vi "EditorPopUp.vi"(8 "error in (no error)":errorcluster, 11 "MAUI.Editor":refnum<class "MAUI.Editor.lvclass">) -> (0 "error out":errorcluster, 3 "MAUI.Editor out":refnum<class "MAUI.Editor.lvclass">)   [LabVIEW 2019, in "MAUI.Editor.lvclass"]
uses:
  MAUI.Editor.lvclass
panel:
  in  "Listbox":i32(listbox)
  in  "Save":bool
  in  "Select":bool
  in  "Refresh":bool
  in  "Configure":bool
  in  "New":bool
  in  "Delete":bool
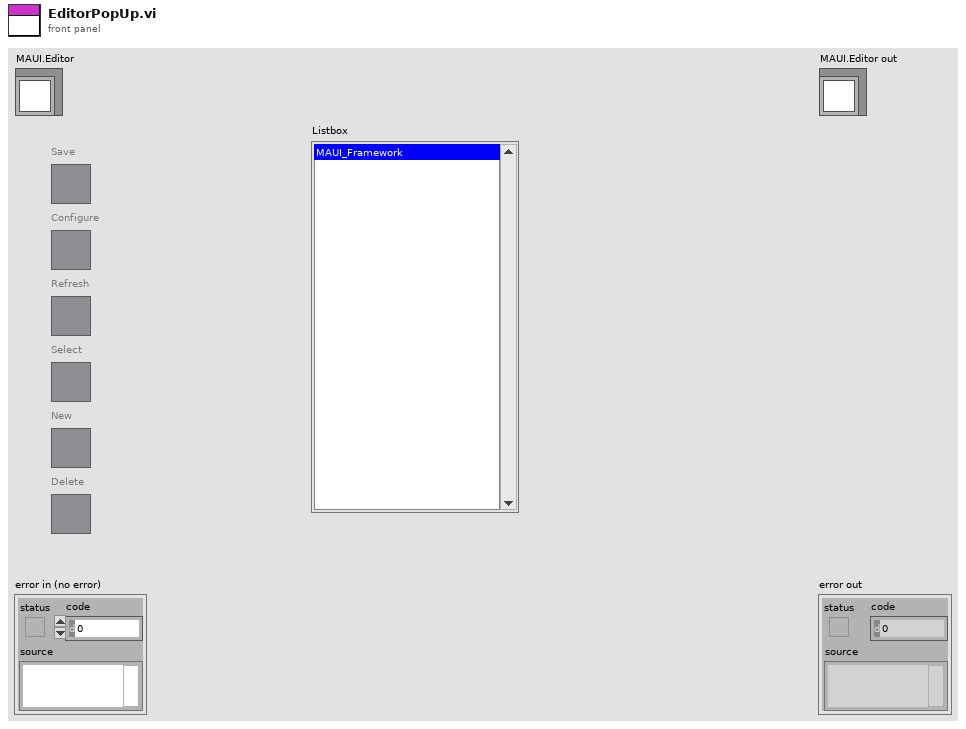
[diagram p1: front panel]
types:
  T1 = enum32{"Invalid", "Standard", "Closed", "Hidden", "Minimized", "Maximized"}
  T2 = enum32{"invalid app kind", "Development System", "Run Time System", "Student Edition", "Embedded LabVIEW", "Evaluation", "Custom"}
  T3 = cluster{"Core":cluster{"Current VI Reference":refnum<vi>, "Close Panel on Exit?":bool}, "MAUI.Editor":refnum<class "MAUI.Editor.lvclass">, "Unsaved?":bool}
  T4 = cluster{"Current VI Reference":refnum<vi>, "Close Panel on Exit?":bool}
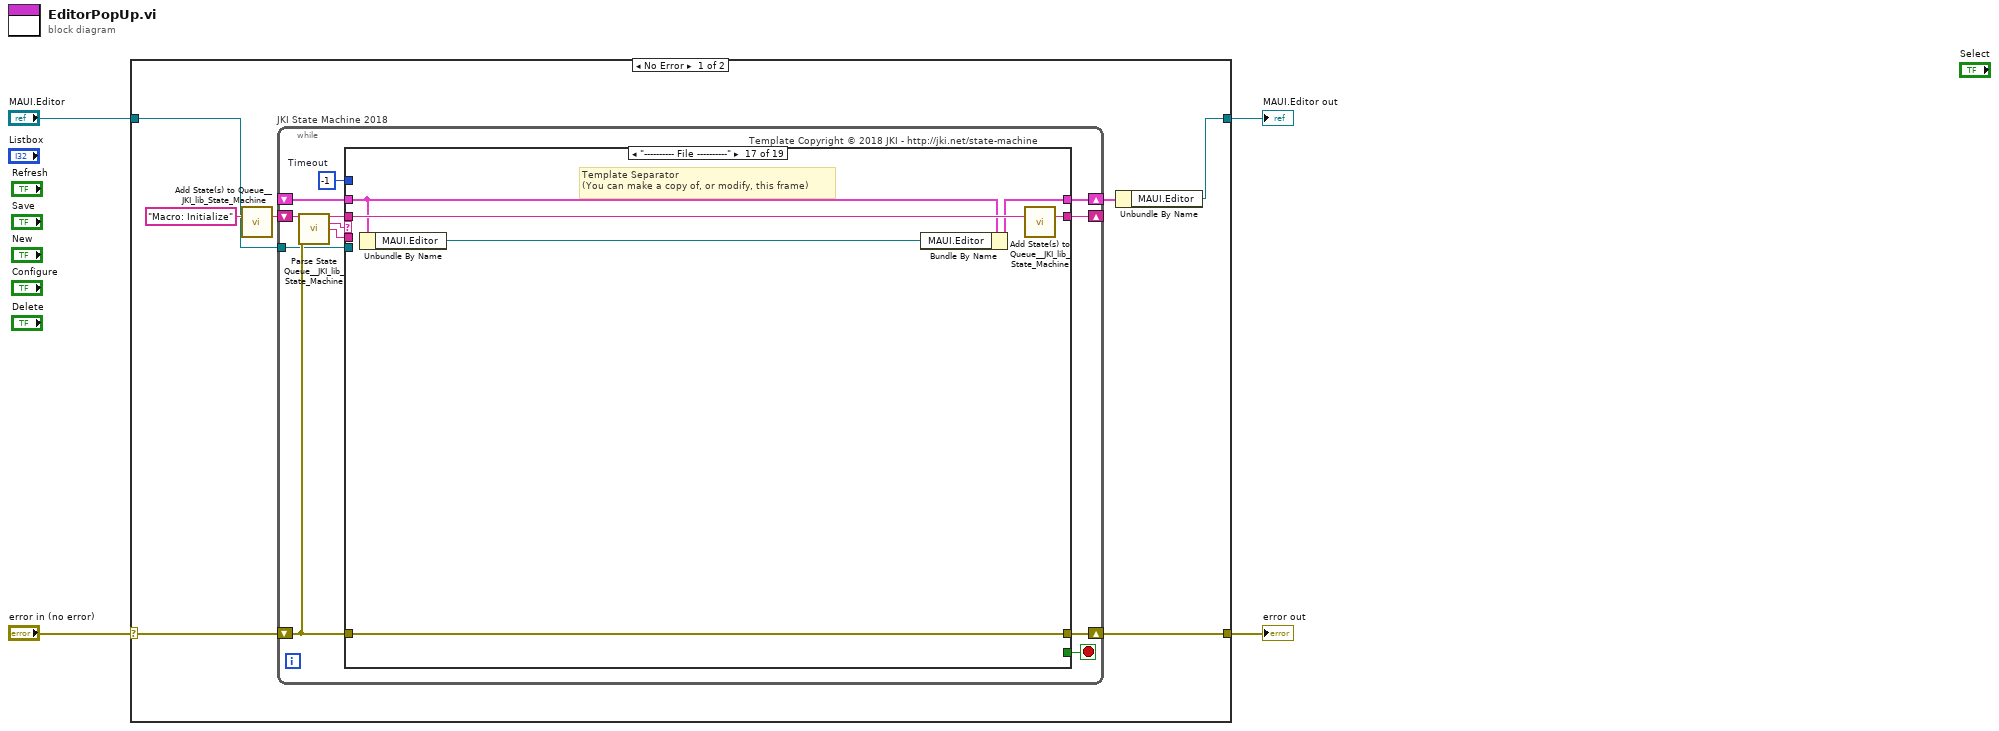
[diagram p0: block diagram]
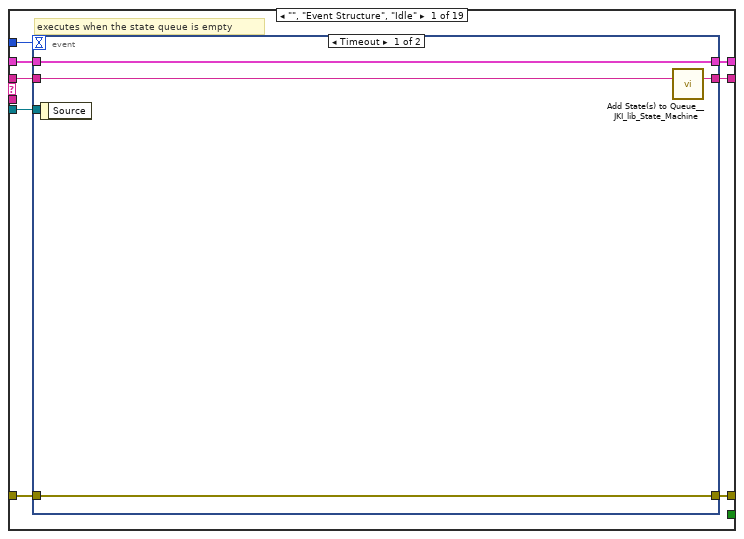
[diagram p2: hidden frame]
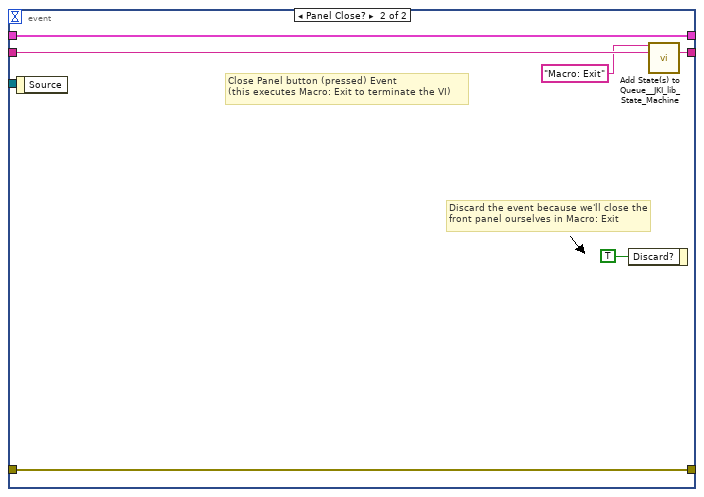
[diagram p3: hidden frame]
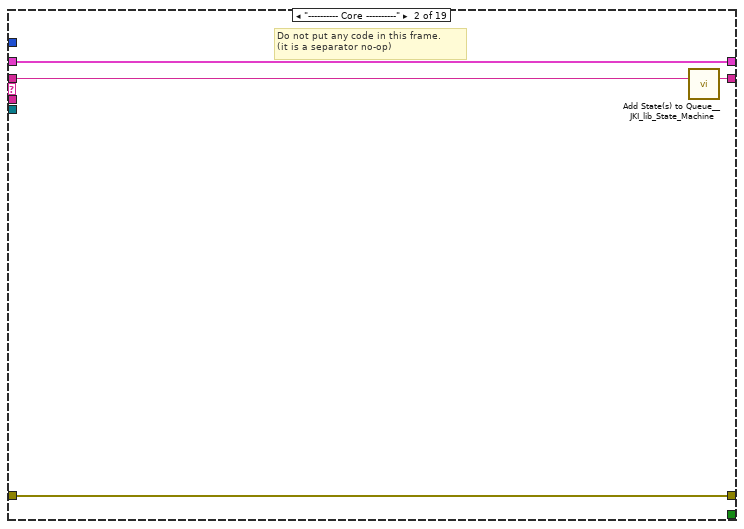
[diagram p4: hidden frame]
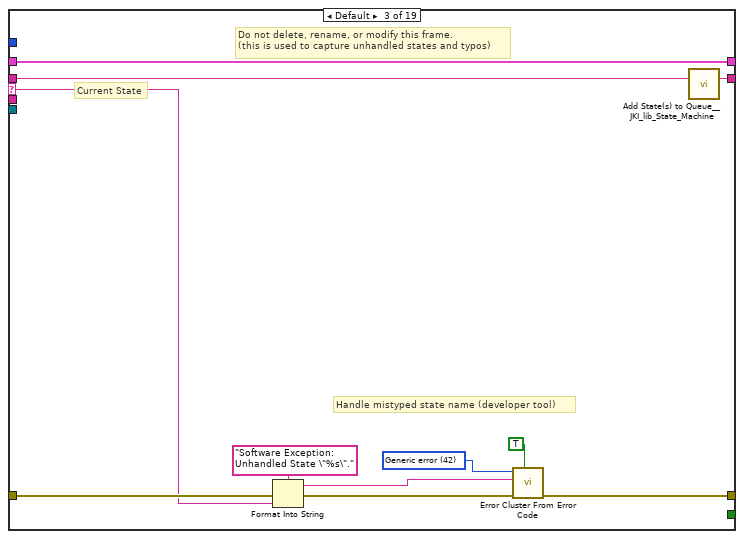
[diagram p5: hidden frame]
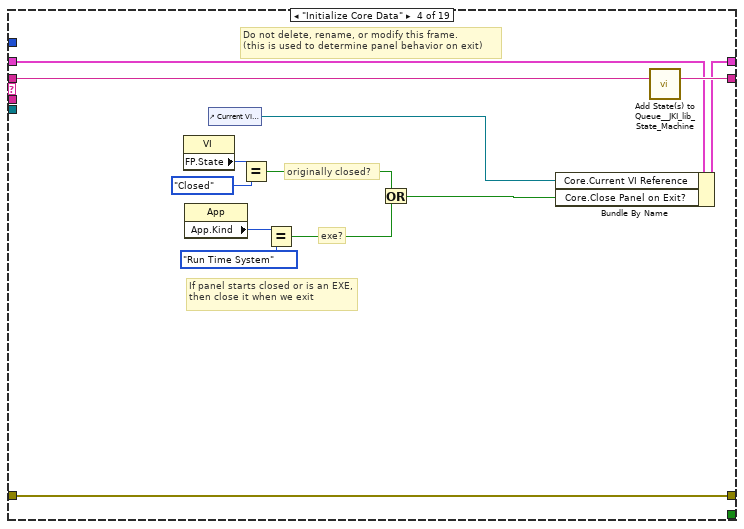
[diagram p6: hidden frame]
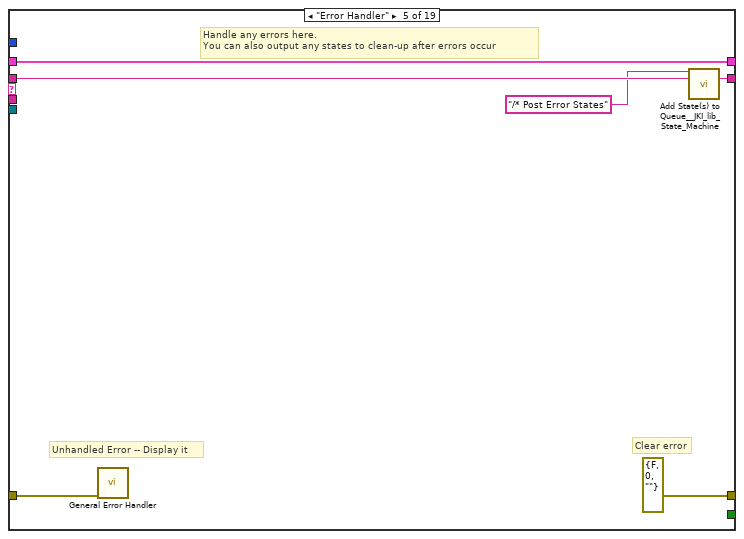
[diagram p7: hidden frame]
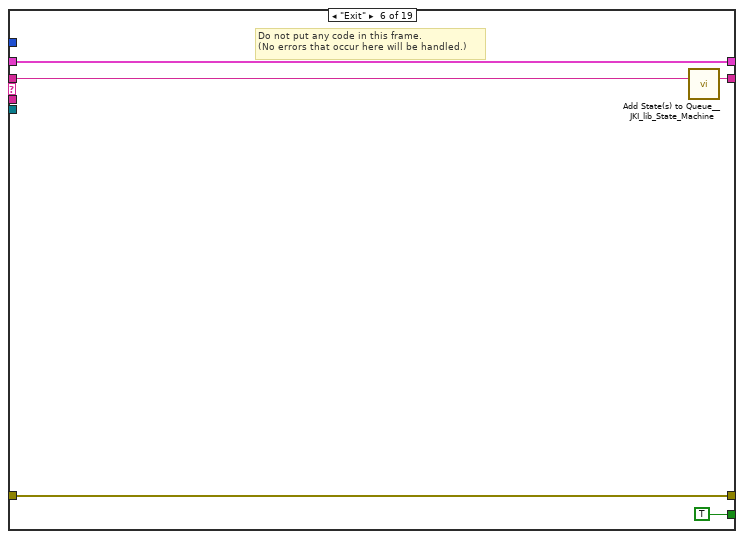
[diagram p8: hidden frame]
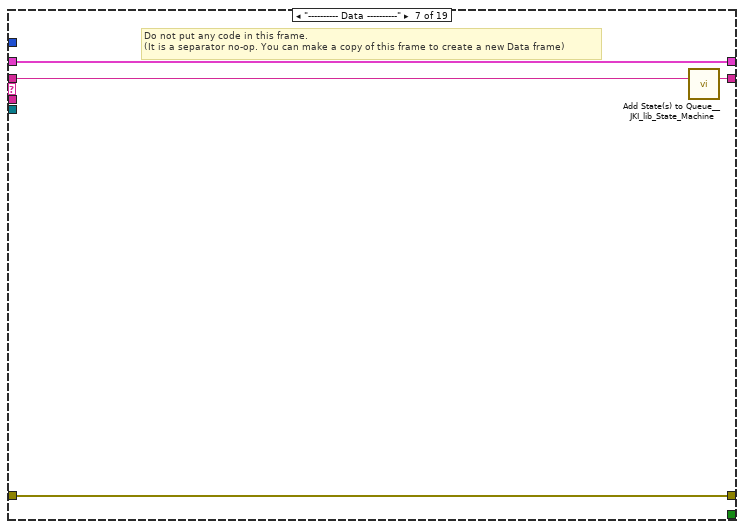
[diagram p9: hidden frame]
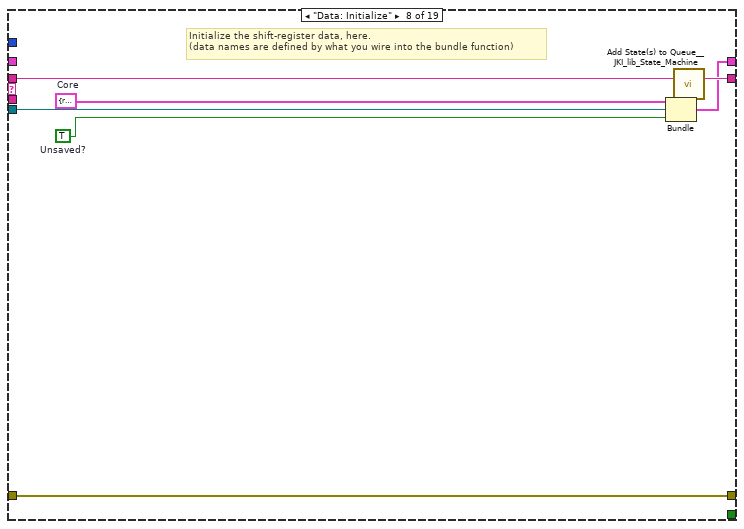
[diagram p10: hidden frame]
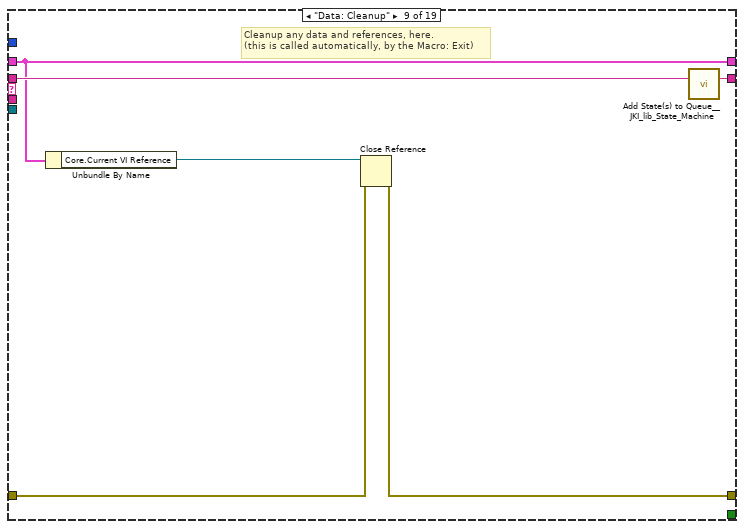
[diagram p11: hidden frame]
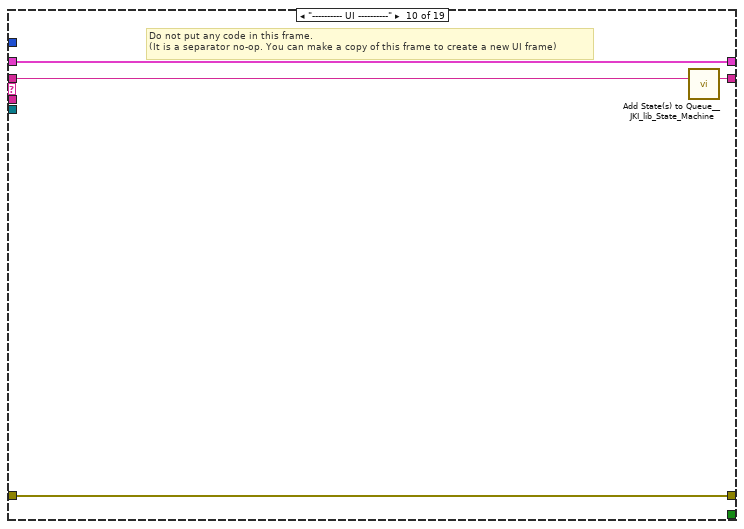
[diagram p12: hidden frame]
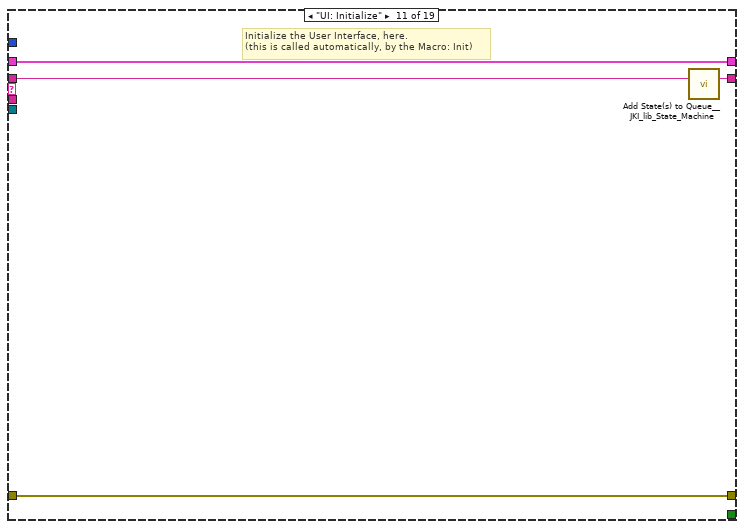
[diagram p13: hidden frame]
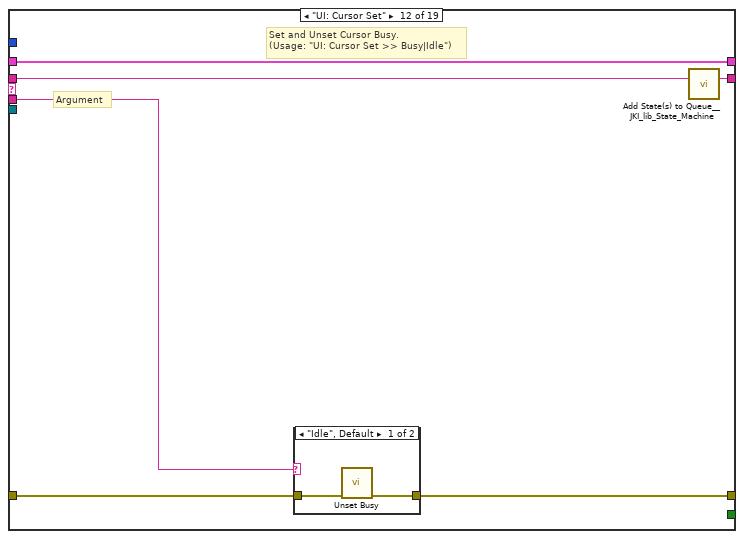
[diagram p14: hidden frame]
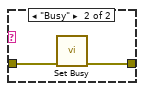
[diagram p15: hidden frame]
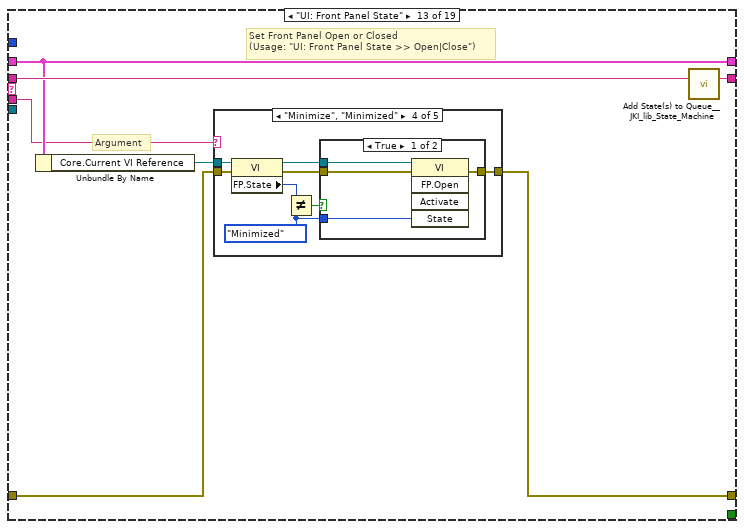
[diagram p16: hidden frame]
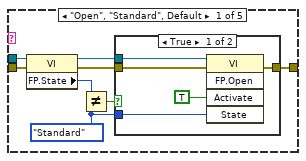
[diagram p17: hidden frame]
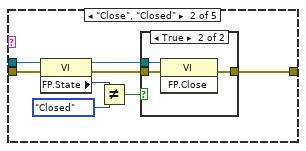
[diagram p19: hidden frame]
diagram:
  n1 = case shown="No Error" "error in (no error)" {
    selector: "error in (no error)" -> [w5 w224]
    tunnel: [w6 w224] -> w3
    tunnel: [w7 w223] -> w1
    tunnel: "MAUI.Editor" -> [w8 w223]
    frame No Error {
      n2 = call <vilib>:"Add State(s) to Queue__JKI_lib_State_Machine.vi"("State(s) in (\"\")"="Macro: Initialize") -> ("States Out"=w11:string)  [unwired: 14 in]
      n3 = while "JKI State Machine 2018" {
        shift-right: [w16] -> w9
        shift-left: _ -> [w15]
        shift-right: [w19] -> w6
        shift-left: w5 -> [w13]
        shift-right: [w18] -> _
        shift-left: w11 -> [w20]
        tunnel: w8 -> [w12]
        stop <- w17 stop-if-true
        w14 = -1  # Timeout
        # "Template Copyright © 2018 JKI - http://jki.net/state-machine"
        n4 = call <vilib>:"Parse State Queue__JKI_lib_State_Machine.vi"("State Queue"=w20, "Error In (no error)"=w13) -> ("Remaining States"=w22:string, "Current State"=w23:string, "Arguments"=w21:string)  [unwired: 11 in]
        n5 = case shown="\"---------- File ----------\"" w23 {
          selector: w23 -> [_ _ w46 _ _ _ _ _ _ _ _ _ _ _ _ _ _ _ _]
          tunnel: w22 -> [w31 w45 w50 w69 w75 w80 w84 w91 w97 w101 w105 w111 w122 w191 w196 w206 w212 w218 w222]
          tunnel: w21 -> [_ _ _ _ _ _ _ _ _ _ _ w106 w116 _ _ _ _ _ _]
          tunnel: w15 -> [w29 w42 w48 w62 w72 w78 w81 _ w92 w98 w103 w109 w118 w188 w193 w203 w208 w214 w220]
          tunnel: [w28 w43 w52 w66 errorcluster {"status"=FALSE, "code"=0, "source"=""} ("error out") w77 w82 w88 w93 w99 w102 w107 w119 w189 w194 w204 w210 w216 w219] -> w19
          tunnel: w13 -> [w27 w43 w51 w66 w71 w77 w82 w88 w94 w99 w102 w108 w120 w189 w194 w204 w210 w216 w219]
          tunnel: [w30 w44 w49 w68 w74 w79 w83 w90 w96 w100 w104 w110 w121 w190 w195 w205 w211 w217 w221] -> w18
          tunnel: [_ _ _ _ _ TRUE _ _ _ _ _ _ _ _ _ _ _ _ _] -> w17
          tunnel: [w26 w42 w48 w67 w72 w78 w81 w89 w92 w98 w103 w109 w118 w188 w193 w203 w209 w215 w220] -> w16
          tunnel: w14 -> [w25 _ _ _ _ _ _ _ _ _ _ _ _ _ _ _ _ _ _]
          tunnel: w12 -> [w24 _ _ _ _ _ _ w86 _ _ _ _ _ _ _ _ _ _ _]
          frame "", "Event Structure", "Idle" {
            # "executes when the state queue is empty"
            n6 = event shown="[0] Timeout" {
              selector: _ -> [_ _]
              dyn-events: _ -> [_ _]
              timeout: w25 -> [_ _]
              tunnel: w31 -> [w35 w41]
              tunnel: [w34 w40] -> w30
              tunnel: w29 -> [w32 w38]
              tunnel: [w33 w39] -> w28
              tunnel: w27 -> [w33 w39]
              tunnel: [w32 w38] -> w26
              tunnel: w24 -> [_ _]
              event Timeout {
                n7 = event-data() -> ()  [unwired: 1 in, 1 out]
                n8 = call <vilib>:"Add State(s) to Queue__JKI_lib_State_Machine.vi"("State(s) in (\"\")"=w35) -> ("States Out"=w34:string)  [unwired: 14 in]
              }
              event Panel Close? {
                # "Discard the event because we'll close the front panel ourselves in Macro: Exit"
                # "Close Panel button (pressed) Event\n(this executes Macro: Exit to terminate the VI)"
                n9 = event-data() -> ()  [unwired: 1 in, 1 out]
                n10 = event-data("Discard?"=TRUE) -> ()  [unwired: 1 in, 1 out]
                n11 = call <vilib>:"Add State(s) to Queue__JKI_lib_State_Machine.vi"("State(s) in Front (\"\")"="Macro: Exit", "State(s) in (\"\")"=w41) -> ("States Out"=w40:string)  [unwired: 13 in]
              }
            }
          }
          frame "---------- Core ----------" {
            # "Do not put any code in this frame.\n(it is a separator no-op)"
            n12 = call <vilib>:"Add State(s) to Queue__JKI_lib_State_Machine.vi"("State(s) in (\"\")"=w45) -> ("States Out"=w44:string)  [unwired: 14 in]
          }
          frame Default {
            w55 = 42 items=["No error", "Argument error", "Memory is full", "Out of zone", "End of file", "File already open", "Generic file I/O error", "File not found", "File permission error", "Disk is full", "Duplicate path", "Too many files open", "System feature not enabled", "Resource file not found", "Cannot add resource", "Resource not found", "Image not found", "Image memory error", "Pen does not exist", "Config type invalid", "Config token not found", "Config parse error", "Config memory error", "Bad external code format", "Bad external code offset", "External code not present", "Null window", "Destroy window error", "Null menu", "Print aborted", "Bad print record", "Print driver error", "Windows error during printing", "Memory error during printing", "Print dialog error", "Generic print error", "Invalid device refnum", "Device not found", "Device parameter error", "Device unit error", "Cannot open device", "Device call aborted", "Generic error", "Cancelled by user", "Object ID too low", "Object ID too high", "Object not in heap", "Unknown heap", "Unknown object (invalid DefProc)", "Unknown object (DefProc not in table)", "Message out of range", "Invalid (null) method", "Unknown message", "Manager call not supported", "Bad address", "Network operation in progress", "Network operation timed out", "Connection is busy", "Network attribute not supported", "Network error", "Address in use", "System out of memory", "Connection aborted", "Connection refused", "Not connected", "Already connected", "Connection closed", "Initialization error (interapplication manager)", "Bad occurrence", "Wait on unbound occurrence handler", "Occurrence queue overflow", "Datalog type conflict", "Unused", "Unrecognized type (interapplication manager)", "Memory corrupt", "Failed to make temporary DLL", "Old CIN version", "Drag socket not found", "Failed to load drop-object", "Failed to register OLE object", "Failed to release OLE object", "Format specifier type mismatch", "Unknown format specifier", "Too few format specifiers", "Too many format specifiers", "Scan failed", "Newer CIN version", "Error converting to variant", "Runtime menu error", "Password tampered", "Variant attribute not found", "Incompatible variant data type", "Event data is not available", "Event Store is not present", "Occurrence is not found", "Event Queue is not created", "Event info is not available", "Refnum passed is NULL", "Error retrieving Class GUID", "Error retrieving CoClass GUID", "Error retrieving TypeLib GUID.", "Bad built application magic bytes.", "Specific driver is different from the specific driver associated with the Logical Name.", "There is no session opened to the class driver.", "Max Error", "MAX - Error with config objects", "MAX - Error loading configuration", "MAX - Group not supported"]
            # "Current State"
            # "Do not delete, rename, or modify this frame.\n(this is used to capture unhandled states and typos)"
            # "Handle mistyped state name (developer tool)"
            n13 = Format Into String(format string="Software Exception: Unhandled State \"%s\"." ("message"), error in=w51, w46) -> (resulting string=w54:string, error out=w53:errorcluster)  [unwired: 1 in]
            n14 = call <vilib>:"Error Cluster From Error Code.vi"("show call chain? (False)"=TRUE, "error in (no error)"=w53, "error message (\"\")"=w54, "error code (0)"=w55) -> ("error out"=w52:errorcluster)  [unwired: 5 in]
            n15 = call <vilib>:"Add State(s) to Queue__JKI_lib_State_Machine.vi"("State(s) in (\"\")"=w50) -> ("States Out"=w49:string)  [unwired: 14 in]
          }
          frame "Initialize Core Data" {
            # "Do not delete, rename, or modify this frame.\n(this is used to determine panel behavior on exit)"
            # "originally closed?"
            # "exe?"
            # "If panel starts closed or is an EXE, then close it when we exit"
            n16 = property class="VI"() -> ("FP.State"=w59:T1)  [unwired: 2 in, 2 out]
            n17 = property class="App"() -> ("App.Kind"=w65:T2)  [unwired: 2 in, 2 out]
            n18 = control-ref of="Current VI Reference"() -> (w60:refnum<vi>)
            n19 = Equal?(x=w59, y=T1."Closed" ("Front Panel Window:State")) -> (x = y?=w57:bool)
            n20 = Equal?(x=w65, y=T2."Run Time System" ("Application:Kind")) -> (x = y?=w63:bool)
            n21 = Or(x=w57, y=w63) -> (x .or. y?=w61:bool)
            n22 = Bundle By Name(cluster=w62, "Core.Current VI Reference"=w60, "Core.Close Panel on Exit?"=w61) -> (w67:T3)
            n23 = call <vilib>:"Add State(s) to Queue__JKI_lib_State_Machine.vi"("State(s) in (\"\")"=w69) -> ("States Out"=w68:string)  [unwired: 14 in]
          }
          frame "Error Handler" {
            # "Unhandled Error -- Display it"
            # "Handle any errors here.\nYou can also output any states to clean-up after errors occur"
            # "Clear error"
            n24 = call <vilib>:"General Error Handler.vi"("error in (no error)"=w71) -> ()  [unwired: 10 in, 5 out]
            n25 = call <vilib>:"Add State(s) to Queue__JKI_lib_State_Machine.vi"("State(s) in Front (\"\")"="/* Post Error States", "State(s) in (\"\")"=w75) -> ("States Out"=w74:string)  [unwired: 13 in]
          }
          frame "Exit" {
            # "Do not put any code in this frame.\n(No errors that occur here will be handled.)"
            n26 = call <vilib>:"Add State(s) to Queue__JKI_lib_State_Machine.vi"("State(s) in (\"\")"=w80) -> ("States Out"=w79:string)  [unwired: 14 in]
          }
          frame "---------- Data ----------" {
            # "Do not put any code in this frame.\n(It is a separator no-op. You can make a copy of this frame to create a new Data frame)"
            n27 = call <vilib>:"Add State(s) to Queue__JKI_lib_State_Machine.vi"("State(s) in (\"\")"=w84) -> ("States Out"=w83:string)  [unwired: 14 in]
          }
          frame "Data: Initialize" {
            w85 = TRUE  # Unsaved?
            w87 = T4 {"Current VI Reference"=refnum, "Close Panel on Exit?"=FALSE}  # Core
            # "Initialize the shift-register data, here.\n(data names are defined by what you wire into the bundle function)"
            n28 = Bundle("Core"=w87, "MAUI.Editor"=w86, "Unsaved?"=w85) -> (w89:T3)  [unwired: 1 in]
            n29 = call <vilib>:"Add State(s) to Queue__JKI_lib_State_Machine.vi"("State(s) in (\"\")"=w91) -> ("States Out"=w90:string)  [unwired: 14 in]
          }
          frame "Data: Cleanup" {
            # "Cleanup any data and references, here.\n(this is called automatically, by the Macro: Exit)"
            n30 = Unbundle By Name(w92) -> ("Core.Current VI Reference"=w95:refnum<vi>)
            n31 = Close Reference(reference=w95, error in (no error)=w94) -> (error out=w93:errorcluster)
            n32 = call <vilib>:"Add State(s) to Queue__JKI_lib_State_Machine.vi"("State(s) in (\"\")"=w97) -> ("States Out"=w96:string)  [unwired: 14 in]
          }
          frame "---------- UI ----------" {
            # "Do not put any code in this frame.\n(It is a separator no-op. You can make a copy of this frame to create a new UI frame)"
            n33 = call <vilib>:"Add State(s) to Queue__JKI_lib_State_Machine.vi"("State(s) in (\"\")"=w101) -> ("States Out"=w100:string)  [unwired: 14 in]
          }
          frame "UI: Initialize" {
            # "Initialize the User Interface, here.\n(this is called automatically, by the Macro: Init)"
            n34 = call <vilib>:"Add State(s) to Queue__JKI_lib_State_Machine.vi"("State(s) in (\"\")"=w105) -> ("States Out"=w104:string)  [unwired: 14 in]
          }
          frame "UI: Cursor Set" {
            # "Argument"
            # "Set and Unset Cursor Busy.\n(Usage: \"UI: Cursor Set >> Busy|Idle\")"
            n35 = case shown="\"Idle\", Default" w106 {
              tunnel: w108 -> [w113 w115]
              tunnel: [w112 w114] -> w107
              frame "Idle", Default {
                n36 = call <vilib>:"Unset Busy.vi"("error in (no error)"=w113) -> ("error out"=w112:errorcluster)  [unwired: 10 in]
              }
              frame "Busy" {
                n37 = call <vilib>:"Set Busy.vi"("error in (no error)"=w115) -> ("error out"=w114:errorcluster)  [unwired: 9 in, 1 out]
              }
            }
            n38 = call <vilib>:"Add State(s) to Queue__JKI_lib_State_Machine.vi"("State(s) in (\"\")"=w111) -> ("States Out"=w110:string)  [unwired: 14 in]
          }
          frame "UI: Front Panel State" {
            # "Argument"
            # "Set Front Panel Open or Closed\n(Usage: \"UI: Front Panel State >> Open|Close\")"
            n39 = Unbundle By Name(w118) -> ("Core.Current VI Reference"=w117:refnum<vi>)
            n40 = case shown="\"Minimize\", \"Minimized\"" w116 {
              tunnel: w120 -> [w128 w143 w154 w167 w180]
              tunnel: [w130 w144 w156 w169 w182] -> w119
              tunnel: w117 -> [w129 w141 w155 w168 w181]
              frame "Open", "Standard", Default {
                w123 = T1."Standard" ("State")
                n41 = property class="VI"(reference=w129, error in=w128) -> (reference out=w126:refnum<vi>, error out=w127:errorcluster, "FP.State"=w125:T1)
                n42 = Not Equal?(x=w125, y=w123) -> (x != y?=w124:bool)
                n43 = case shown="True" w124 {
                  tunnel: [w134 w136] -> w130
                  tunnel: w127 -> [w133 w136]
                  tunnel: w126 -> [w132 _]
                  tunnel: w123 -> [w131 _]
                  frame True {
                    n44 = invoke class="VI" method="FP.Open"(reference=w132, error in=w133, "Activate"=TRUE, "State"=w131) -> (error out=w134:errorcluster)  [unwired: 1 in, 4 out]
                  }
                  frame False {
                  }
                }
              }
              frame "Close", "Closed" {
                n45 = property class="VI"(reference=w141, error in=w143) -> (reference out=w140:refnum<vi>, error out=w142:errorcluster, "FP.State"=w138:T1)
                n46 = Not Equal?(x=w138, y=T1."Closed" ("Front Panel Window:State")) -> (x != y?=w137:bool)
                n47 = case shown="True" w137 {
                  tunnel: [w145 w148] -> w144
                  tunnel: w142 -> [w145 w147]
                  tunnel: w140 -> [_ w146]
                  frame False {
                  }
                  frame True {
                    n48 = invoke class="VI" method="FP.Close"(reference=w146, error in=w147) -> (error out=w148:errorcluster)  [unwired: 1 in, 2 out]
                  }
                }
              }
              frame "Hidden", "Hide" {
                w149 = T1."Hidden" ("State")
                n49 = property class="VI"(reference=w155, error in=w154) -> (reference out=w152:refnum<vi>, error out=w153:errorcluster, "FP.State"=w151:T1)
                n50 = Not Equal?(x=w151, y=w149) -> (x != y?=w150:bool)
                n51 = case shown="True" w150 {
                  tunnel: [w160 w161] -> w156
                  tunnel: w153 -> [w159 w161]
                  tunnel: w152 -> [w158 _]
                  tunnel: w149 -> [w157 _]
                  frame True {
                    n52 = invoke class="VI" method="FP.Open"(reference=w158, error in=w159, "State"=w157) -> (error out=w160:errorcluster)  [unwired: 2 in, 4 out]
                  }
                  frame False {
                  }
                }
              }
              frame "Minimize", "Minimized" {
                w162 = T1."Minimized" ("State")
                n53 = property class="VI"(reference=w168, error in=w167) -> (reference out=w165:refnum<vi>, error out=w166:errorcluster, "FP.State"=w164:T1)
                n54 = Not Equal?(x=w164, y=w162) -> (x != y?=w163:bool)
                n55 = case shown="True" w163 {
                  tunnel: [w173 w174] -> w169
                  tunnel: w166 -> [w172 w174]
                  tunnel: w165 -> [w171 _]
                  tunnel: w162 -> [w170 _]
                  frame True {
                    n56 = invoke class="VI" method="FP.Open"(reference=w171, error in=w172, "State"=w170) -> (error out=w173:errorcluster)  [unwired: 2 in, 4 out]
                  }
                  frame False {
                  }
                }
              }
              frame "Maximize", "Maximized" {
                w175 = T1."Maximized" ("State")
                n57 = property class="VI"(reference=w181, error in=w180) -> (reference out=w178:refnum<vi>, error out=w179:errorcluster, "FP.State"=w177:T1)
                n58 = Not Equal?(x=w177, y=w175) -> (x != y?=w176:bool)
                n59 = case shown="True" w176 {
                  tunnel: [w186 w187] -> w182
                  tunnel: w179 -> [w185 w187]
                  tunnel: w178 -> [w184 _]
                  tunnel: w175 -> [w183 _]
                  frame True {
                    n60 = invoke class="VI" method="FP.Open"(reference=w184, error in=w185, "State"=w183) -> (error out=w186:errorcluster)  [unwired: 2 in, 4 out]
                  }
                  frame False {
                  }
                }
              }
            }
            n61 = call <vilib>:"Add State(s) to Queue__JKI_lib_State_Machine.vi"("State(s) in (\"\")"=w122) -> ("States Out"=w121:string)  [unwired: 14 in]
          }
          frame "---------- Macro ----------" {
            # "Do not put any code in this frame.\n(It is a separator no-op. You can make a copy of this frame to create a new Macro frame)"
            n62 = call <vilib>:"Add State(s) to Queue__JKI_lib_State_Machine.vi"("State(s) in (\"\")"=w191) -> ("States Out"=w190:string)  [unwired: 14 in]
          }
          frame "Macro: Initialize" {
            w192 = "Data: Initialize\nInitialize Core Data\nUI: Initialize\nUI: Front Panel State >> Open\nEditor: Find Applications"  # Data: Initialize Initialize Core Data UI: Initialize UI: Front Panel State >> Open Editor: Find Applications
            # "Initialization Macro\n(This is called once, when the VI starts)"
            n63 = call <vilib>:"Add State(s) to Queue__JKI_lib_State_Machine.vi"("State(s) in Front (\"\")"=w192, "State(s) in (\"\")"=w196) -> ("States Out"=w195:string)  [unwired: 13 in]
          }
          frame "Macro: Exit" {
            # "Exit Macro\n(This is called once, when the VI exits)"
            n64 = Unbundle By Name(w203) -> ("Core.Close Panel on Exit?"=w202:bool)
            n65 = Select(t="UI: Front Panel State >> Close", s=w202, f="") -> (s? t:f=w199:string)
            n66 = call <vilib>:"Add State(s) to Queue__JKI_lib_State_Machine.vi"("State(s) in (\"\")"=w199, "State(s) at Back (\"\")"="Data: Cleanup\nExit") -> ("States Out"=w197:string)  [unwired: 13 in]
            n67 = call <vilib>:"Add State(s) to Queue__JKI_lib_State_Machine.vi"("State(s) in Front (\"\")"=w197, "State(s) in (\"\")"=w206) -> ("States Out"=w205:string)  [unwired: 13 in]
          }
          frame "---------- File ----------" {
            # "Template Separator\n(You can make a copy of, or modify, this frame)"
            n68 = Unbundle By Name(w208) -> ("MAUI.Editor"=w207:refnum<class "MAUI.Editor.lvclass">)
            n69 = Bundle By Name(cluster=w208, "MAUI.Editor"=w207) -> (w209:T3)
            n70 = call <vilib>:"Add State(s) to Queue__JKI_lib_State_Machine.vi"("State(s) in (\"\")"=w212) -> ("States Out"=w211:string)  [unwired: 14 in]
          }
          frame "---------- Editor ----------" {
            # "Template Separator\n(You can make a copy of, or modify, this frame)"
            n71 = Unbundle By Name(w214) -> ("MAUI.Editor"=w213:refnum<class "MAUI.Editor.lvclass">)
            n72 = Bundle By Name(cluster=w214, "MAUI.Editor"=w213) -> (w215:T3)
            n73 = call <vilib>:"Add State(s) to Queue__JKI_lib_State_Machine.vi"("State(s) in (\"\")"=w218) -> ("States Out"=w217:string)  [unwired: 14 in]
          }
          frame "Editor: Find Applications" {
            # "Template Separator\n(You can make a copy of, or modify, this frame)"
            n74 = call <vilib>:"Add State(s) to Queue__JKI_lib_State_Machine.vi"("State(s) in (\"\")"=w222) -> ("States Out"=w221:string)  [unwired: 14 in]
          }
        }
      }
      n75 = Unbundle By Name(w9) -> ("MAUI.Editor"=w7:refnum<class "MAUI.Editor.lvclass">)
    }
    frame Error {
    }
  }
  "error out" <- w3
  "MAUI.Editor out" <- w1
